vi "Register Sessions Wrapper.vi"(8 "error in":errorcluster, 11 "request data":T2) -> (0 "error out":errorcluster, 3 "response data":T1)   [LabVIEW 2020, in "NI Session Management V1 Client.lvlib" / "Session Reservation.lvclass"]
uses:
  Session Reservation.lvclass
  gRPC/Generated APIs/ni/measurementlink/sessionmanagement/v1/RPC Messages/ni_measurementlink_sessionmanagement_v1_RegisterSessionsRequest.ctl
  gRPC/Generated APIs/ni/measurementlink/sessionmanagement/v1/RPC Messages/ni_measurementlink_sessionmanagement_v1_SessionInformation.ctl
  gRPC/Generated APIs/ni/measurementlink/sessionmanagement/v1/RPC Messages/nidevice_grpc_Session.ctl
  gRPC/Generated APIs/ni/measurementlink/sessionmanagement/v1/RPC Messages/ni_measurementlink_sessionmanagement_v1_ChannelMapping.ctl
  gRPC/Generated APIs/ni/measurementlink/sessionmanagement/v1/RPC Messages/ni_measurementlink_sessionmanagement_v1_RegisterSessionsResponse.ctl
  Discovery V1/TypeDefs/gRPC Client Cache FGV Action.ctl
  Discovery V1/NI Discovery V1 Client.lvlib
  gRPC/Generated APIs/ni/measurementlink/sessionmanagement/v1/ni.measurementlink.sessionmanagement.v1.api.lvlib
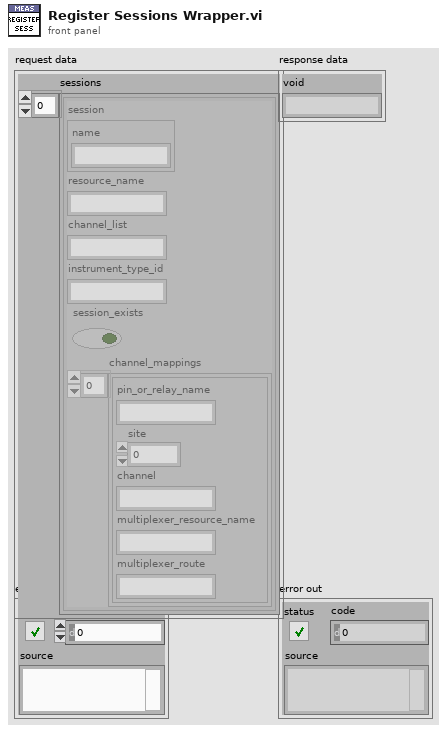
[diagram p1: front panel]
types:
  T1 = typedef "ni.measurementlink.sessionmanagement.v1.api.lvlib/ni_measurementlink_sessionmanagement_v1_RegisterSessionsResponse.ctl" = cluster{"void":string}
  T2 = typedef "ni.measurementlink.sessionmanagement.v1.api.lvlib/ni_measurementlink_sessionmanagement_v1_RegisterSessionsRequest.ctl" = cluster{"sessions":T3[]}
  T3 = typedef "ni.measurementlink.sessionmanagement.v1.api.lvlib/ni_measurementlink_sessionmanagement_v1_SessionInformation.ctl" = cluster{"session":T4, "resource_name":string, "channel_list":string, "instrument_type_id":string, "session_exists":bool, "channel_mappings":T5[]}
  T4 = typedef "ni.measurementlink.sessionmanagement.v1.api.lvlib/nidevice_grpc_Session.ctl" = cluster{"name":string}
  T5 = typedef "ni.measurementlink.sessionmanagement.v1.api.lvlib/ni_measurementlink_sessionmanagement_v1_ChannelMapping.ctl" = cluster{"pin_or_relay_name":string, "site":i32, "channel":string, "multiplexer_resource_name":string, "multiplexer_route":string}
  T6 = typedef "NI Discovery V1 Client.lvlib/gRPC Client Cache FGV Action.ctl" = enum16{"Get Client", "Recreate Client", "Destroy Client", "Update ClusterId"}
  T7 = typedef "grpc-lvsupport-release.lvlib/grpcId.ctl" = u64
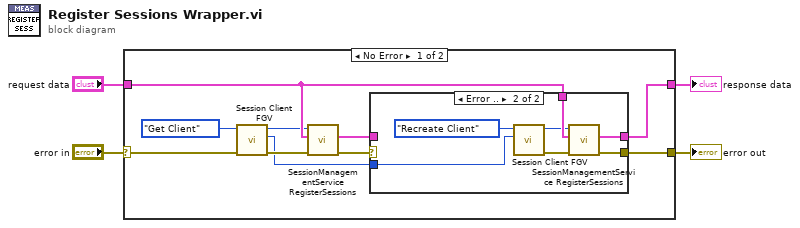
[diagram p0: block diagram]
diagram:
  n1 = case shown="No Error" "error in" {
    selector: "error in" -> [w14 w24]
    tunnel: [w11 w24] -> w3
    tunnel: "request data" -> [w8 _]
    tunnel: [w10 _] -> w1
    frame No Error {
      n2 = call "Session Client FGV.vi"("error in"=w14, "action"=gRPC_Client_Cache_FGV_Action."Get Client") -> ("error out"=w13:errorcluster, "unique id out"=w5:u64, "grpc client id"=w6:T7)  [unwired: 7 in]
      n3 = call "SessionManagementService RegisterSessions.vi"("error in"=w13, "Request Data"=w8, "gRPC ID"=w6) -> ("error out"=w12:errorcluster, "Response Data"=w9:T1)  [unwired: 6 in, 1 out]
      n4 = case shown="Error .." w12 {
        selector: w12 -> [w16 _]
        tunnel: [w16 w22] -> w11
        tunnel: [w15 w21] -> w10
        tunnel: w9 -> [w15 _]
        tunnel: w8 -> [_ w20]
        tunnel: w5 -> [_ w18]
        frame No Error {
        }
        frame Error {
          n5 = call "Session Client FGV.vi"("unique id in"=w18, "action"=gRPC_Client_Cache_FGV_Action."Recreate Client") -> ("error out"=w23:errorcluster, "grpc client id"=w17:T7)  [unwired: 7 in, 1 out]
          n6 = call "SessionManagementService RegisterSessions.vi"("error in"=w23, "Request Data"=w20, "gRPC ID"=w17) -> ("error out"=w22:errorcluster, "Response Data"=w21:T1)  [unwired: 6 in, 1 out]
        }
      }
    }
    frame Error {
    }
  }
  "error out" <- w3
  "response data" <- w1
